vi "test 4.vi"(11 "Match Cluster":T1) -> (3 "csv array":string[][](array[string]))   [LabVIEW 2015]
uses:
  Typedef/JSONCluster.ctl
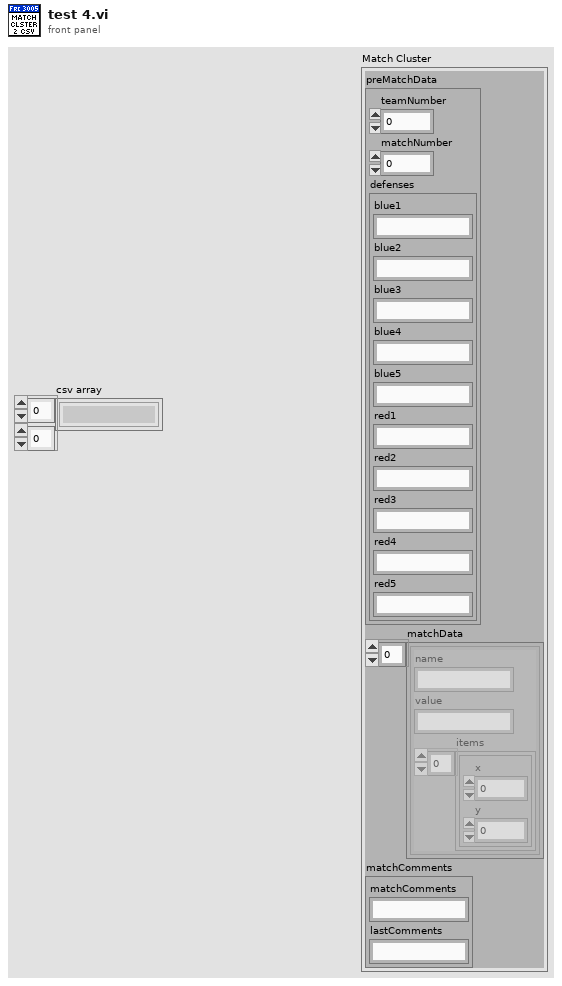
[diagram p1: front panel]
types:
  T1 = typedef "JSONCluster.ctl" = cluster{"preMatchData":cluster{"teamNumber":i32, "matchNumber":i32, "defenses":cluster{"blue1":string, "blue2":string, "blue3":string, "blue4":string, "blue5":string, "red1":string, "red2":string, "red3":string, "red4":string, "red5":string}}, "matchData":cluster{"name":string, "value":string, "items":cluster{"x":i32, "y":i32}[]}[], "matchComments":cluster{"matchComments":string, "lastComments":string}}
  T2 = cluster{"teamNumber":i32, "matchNumber":i32, "defenses":cluster{"blue1":string, "blue2":string, "blue3":string, "blue4":string, "blue5":string, "red1":string, "red2":string, "red3":string, "red4":string, "red5":string}}
  T3 = cluster{"name":string, "value":string, "items":cluster{"x":i32, "y":i32}[]}[]
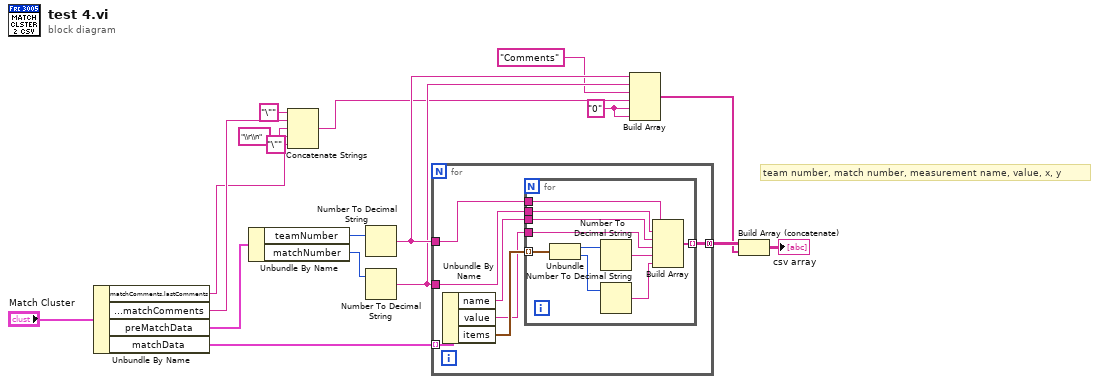
[diagram p0: block diagram]
diagram:
  w7 = "0" ("element")
  # "team number, match number, measurement name, value, x, y"
  n1 = Unbundle By Name("Match Cluster") -> ("matchComments.lastComments"=w9:string, "matchComments.matchComments"=w10:string, "preMatchData"=w17:T2, "matchData"=w18:T3)
  n2 = Unbundle By Name(w17) -> ("teamNumber"=w16:i32, "matchNumber"=w15:i32)
  n3 = Concatenate Strings("\"" ("string"), w10, "\\r\\n" ("string"), w9, "\"" ("string")) -> (w8:string)
  n4 = Number To Decimal String(number=w16) -> (decimal integer string=w14:string)  [unwired: 1 in]
  n5 = Number To Decimal String(number=w15) -> (decimal integer string=w13:string)  [unwired: 1 in]
  n6 = for {
    tunnel: w18 -> [w25] mode=indexing
    tunnel: w14 -> [w21]
    tunnel: w13 -> [w20]
    tunnel: [w19] -> w6 mode=concatenating
    n7 = Unbundle By Name(w25) -> ("name"=w23:string, "value"=w22:string, "items"=w24:cluster{"x":i32, "y":i32}[])
    n8 = for {
      tunnel: w24 -> [w35] mode=indexing
      tunnel: w23 -> [w29]
      tunnel: w22 -> [w30]
      tunnel: w21 -> [w28]
      tunnel: w20 -> [w27]
      tunnel: [w26] -> w19 mode=indexing
      n9 = Unbundle(w35) -> ("x"=w34:i32, "y"=w33:i32)
      n10 = Number To Decimal String(number=w34) -> (decimal integer string=w31:string)  [unwired: 1 in]
      n11 = Number To Decimal String(number=w33) -> (decimal integer string=w32:string)  [unwired: 1 in]
      n12 = Build Array(w28, w27, w29, w30, w31, w32) -> (w26:string[])
    }
  }
  n13 = Build Array(w14, w13, "Comments" ("element"), w8, w7, w7) -> (w5:string[])
  n14 = Build Array (concatenate)(w6, w5) -> (→"csv array":string[][])
